vi "Interpolate 2D.vi"(9 "X":dbl[](array[numeric]), 10 "xi":dbl[](array[numeric]), 11 "2D Array":dbl[][](array[numeric])) -> (3 "yi":dbl[][](array[numeric]))   [LabVIEW 2020]
uses:
  <vilib>/gmath/NI_Gmath.lvlib
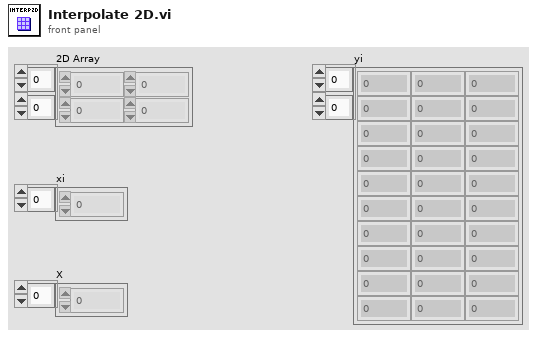
[diagram p1: front panel]
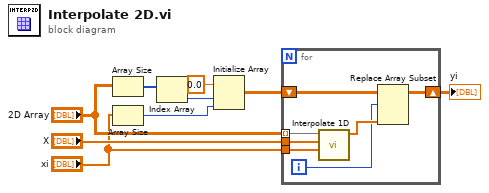
[diagram p0: block diagram]
diagram:
  n1 = Array Size(array="2D Array") -> (size(s)=w7:i32[])
  n2 = Array Size(array="xi") -> (size(s)=w3:i32)
  n3 = Index Array(array=w7) -> (element=w6:i32)  [unwired: 1 in]
  n4 = Initialize Array(0.0 ("element"), w6, w3) -> (w2:dbl[][])
  n5 = for {
    tunnel: "X" -> [w16]
    tunnel: "xi" -> [w15]
    tunnel: "2D Array" -> [w14] mode=indexing
    shift-right: [w11] -> w1
    shift-left: w2 -> [w13]
    i -> [w10]
    n6 = call <vilib>:"Interpolate 1D.vi"("xi"=w15, "X"=w16, "Y"=w14) -> ("yi"=w12:dbl[])  [unwired: 6 in, 2 out]
    n7 = Replace Array Subset(array=w13, new element=w12, index (row)=w10) -> (w11:dbl[][])  [unwired: 1 in]
  }
  "yi" <- w1
